vi "isRunning.vi"(6 "error in (no error)":errorcluster, 7 "fractional run \nthreshold":dbl=0.1, 8 "lower\nspeed bound":dbl=2.4 format="%#_13g", 9 "upper\nspeed bound":dbl=2.7 format="%#_13g", 10 "sample\nlength (ms)":i32=1000, 11 "ballspeed":dbl) -> (3 "isRunning?":bool, 4 "error out":errorcluster)   [LabVIEW 2017]
uses:
  <vilib>/Analysis/baseanly.llb/Mean (DBL).vi
  <vilib>/ptbypt/NI_PtbyPt.lvlib
  <vilib>/Analysis/NI_AALBase.lvlib
panel:
  out "mean ball \nmovement":dbl format="%0.2f"
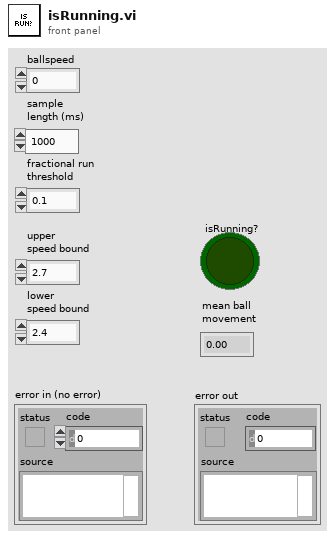
[diagram p1: front panel]
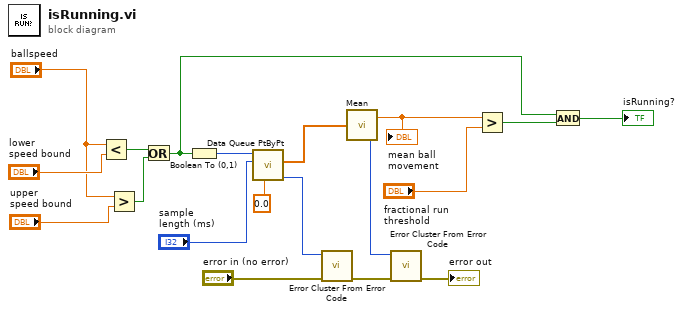
[diagram p0: block diagram]
diagram:
  n1 = Less?(x="ballspeed", y="lower\nspeed bound") -> (x < y?=w17:bool)
  n2 = Greater?(x="ballspeed", y="upper\nspeed bound") -> (0:w16:bool)
  n3 = Or(x=w17, y=w16) -> (x .or. y?=w1:bool)
  n4 = Boolean To (0,1)(Boolean=w1) -> (0, 1=w15:i16)
  n5 = call <vilib>:"Data Queue PtByPt.vi"("initial queue element"=0.0, "sample length"="sample\nlength (ms)", "input data point"=w15) -> ("error"=w12:i32, "Current Queue"=w11:dbl[])  [unwired: 4 in, 3 out]
  n6 = call <vilib>:"Error Cluster From Error Code.vi"("error in (no error)"="error in (no error)", "error code (0)"=w12) -> ("error out"=w7:errorcluster)  [unwired: 7 in]
  n7 = call-poly <vilib>:"Mean.vi"("X"=w11) -> ("mean"=w10:dbl, "error"=w8:i32)
  "mean ball \nmovement" <- w10
  n8 = call <vilib>:"Error Cluster From Error Code.vi"("error in (no error)"=w7, "error code (0)"=w8) -> ("error out"=→"error out":errorcluster)  [unwired: 7 in]
  n9 = Greater?(x=w10, y="fractional run \nthreshold") -> (0:w3:bool)
  n10 = And(x=w1, y=w3) -> (x .and. y?=→"isRunning?":bool)
